vi "Align Mask and Signal - cluster.vi"(0 "Waveform":waveform(dbl)={"t0"=timestamp(0 s since 1904-01-01), "dt"=0.0, "Y"=[]}, 5 "trigger index":i32, 7 "upper limit":cluster{"x0":dbl, "dx":dbl, "Y":dbl[]} {"Y" format="%.2f"; "dx" format="%.2f"; "x0" format="%.2f"}, 9 "lower limit":cluster{"x0":dbl, "dx":dbl, "Y":dbl[]} {"Y" format="%.2f"; "dx" format="%.2f"; "x0" format="%.2f"}, 11 "error in (no error)":errorcluster, 12 "Mask Selector":u16(ring) items=["ITU", "EIA/TIA 547-1989"]) -> (3 "Subset Waveform":waveform(dbl), 4 "Waveform out":waveform(dbl), 6 "upper limit out":cluster{"x0":dbl, "dx":dbl, "Y":dbl[]} {"Y" format="%.2f"; "dx" format="%.2f"; "x0" format="%.2f"}, 8 "lower limit out":cluster{"x0":dbl, "dx":dbl, "Y":dbl[]} {"Y" format="%.2f"; "dx" format="%.2f"; "x0" format="%.2f"}, 15 "error out":errorcluster)   [LabVIEW 2012]
uses:
  <vilib>/Waveform/WDTOps.llb/WDT Number of Waveform Samples DBL.vi
  <vilib>/Waveform/WDTOps.llb/WDT Get Waveform Subset DBL (LV80).vi
  <vilib>/Waveform/WDTOps.llb/WDT Align Waveform Timestamps DBL.vi
  <vilib>/Analysis/NI_AALBase.lvlib
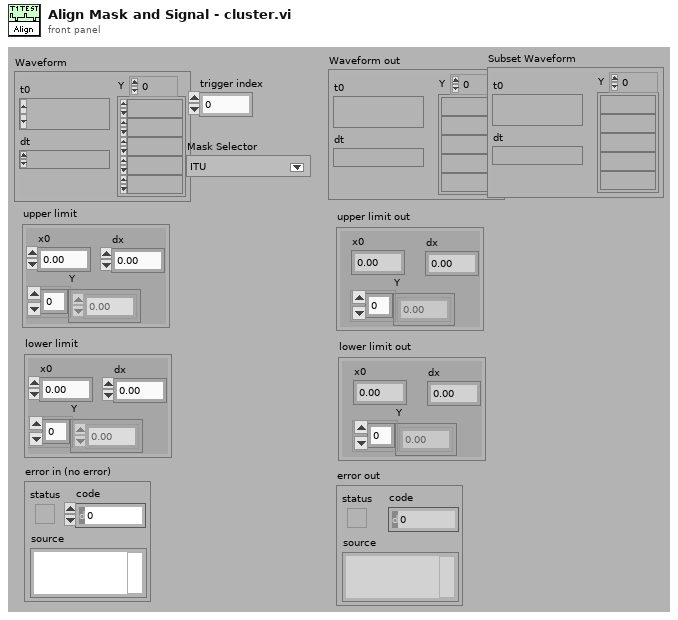
[diagram p1: front panel]
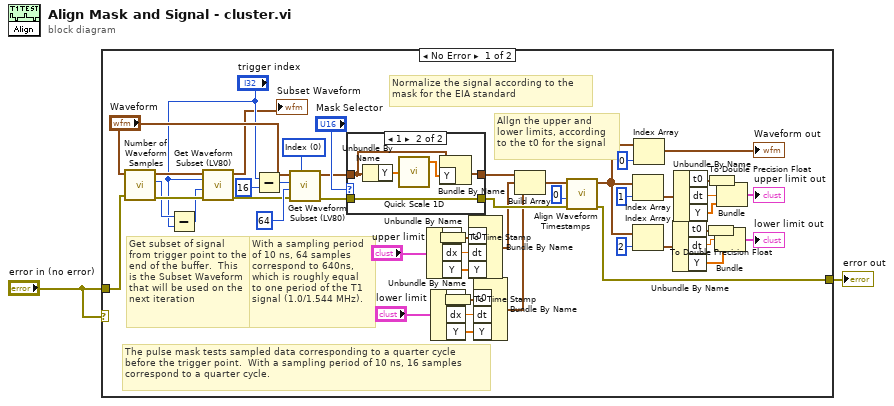
[diagram p0: block diagram]
diagram:
  n1 = case shown="No Error" "error in (no error)" {
    tunnel: "error in (no error)" -> [w39 w60]
    tunnel: [w45 w60] -> w1
    frame No Error {
      w40 = u16 0 items=["Index", "Relative Time"] ("Mode")
      # "Normalize the signal according to the \nmask for the EIA standard"
      # "Allgn the upper and \nlower limits, according \nto the t0 for the signal"
      # "The pulse mask tests sampled data corresponding to a quarter cycle\nbefore the trigger point.  With a sampling period of 10 ns, 16 samples \ncorrespond to a quarter cycle."
      # "With a sampling period\nof 10 ns, 64 samples\ncorrespond to 640ns, \nwhich is roughly equal \nto one period of the T1 \nsignal (1.0/1.544 MHz)."
      # "Get subset of signal\nfrom trigger point to the\nend of the buffer.  This\nis the Subset Waveform\nthat will be used on the \nnext iteration"
      n2 = call-poly <vilib>:"Number of Waveform Samples.vi"("error in (no error)"=w39, "waveform in"="Waveform") -> ("error out"=w37:errorcluster, "number of samples"=w35:i32, "waveform out"=w38:waveform(dbl))  [unwired: 7 in]
      n3 = Subtract(x=w35, y="trigger index") -> (x-y=w33:i32)
      n4 = call-poly <vilib>:"Get Waveform Subset (LV80).vi"("error in (no error)"=w37, "duration"=w33, "start samples/time"="trigger index", "waveform in"=w38) -> ("error out"=w36:errorcluster, "waveform out"=→"Subset Waveform":waveform(dbl))  [unwired: 2 in, 2 out]
      n5 = Subtract(x="trigger index", y=16) -> (x-y=w43:i32)
      n6 = call-poly <vilib>:"Get Waveform Subset (LV80).vi"("start/duration format"=w40, "error in (no error)"=w36, "duration"=64 ("Array Length"), "start samples/time"=w43, "waveform in"="Waveform") -> ("error out"=w30:errorcluster, "waveform out"=w28:waveform(dbl))  [unwired: 1 in, 2 out]
      n7 = case shown="1" "Mask Selector" {
        tunnel: w30 -> [w54 w59]
        tunnel: [w54 w59] -> w29
        tunnel: w28 -> [w53 w57]
        tunnel: [w53 w55] -> w27
        frame 0, Default {
        }
        frame 1 {
          n8 = Unbundle By Name(w57) -> ("Y"=w58:dbl[])
          n9 = call <vilib>:"Quick Scale 1D.vi"("X"=w58) -> ("Y[i]=X[i]/Max|X|"=w56:dbl[])  [unwired: 2 out]
          n10 = Bundle By Name(cluster=w57, "Y"=w56) -> (w55:waveform(dbl))
        }
      }
      n11 = Unbundle By Name("upper limit") -> ("x0"=w25:dbl, "dx"=w24:dbl, "Y"=w23:dbl[])
      n12 = Unbundle By Name("lower limit") -> ("x0"=w18:dbl, "dx"=w20:dbl, "Y"=w21:dbl[])
      n13 = To Time Stamp(1:w25) -> (0:w3:timestamp)
      n14 = To Time Stamp(1:w18) -> (0:w4:timestamp)
      n15 = Bundle By Name("t0"=w3, "dt"=w24, "Y"=w23) -> (w22:waveform(dbl))  [unwired: 1 in]
      n16 = Bundle By Name("t0"=w4, "dt"=w20, "Y"=w21) -> (w17:waveform(dbl))  [unwired: 1 in]
      n17 = Build Array(w27, w22, w17) -> (w52:waveform(dbl)[])
      n18 = call-poly <vilib>:"Align Waveform Timestamps.vi"("error in (no error)"=w29, "index"=0 ("Index"), "waveforms in"=w52) -> ("error out"=w45:errorcluster, "waveforms out"=w50:waveform(dbl)[])  [unwired: 7 in]
      n19 = Index Array(array=w50, index=1 ("Index")) -> (element=w16:waveform(dbl))
      n20 = Index Array(array=w50, index=2 ("Index")) -> (element=w11:waveform(dbl))
      n21 = Index Array(array=w50, index=0 ("Index")) -> (element=→"Waveform out":waveform(dbl))
      n22 = Unbundle By Name(w11) -> ("t0"=w6:timestamp, "dt"=w9:dbl, "Y"=w8:dbl[])
      n23 = Unbundle By Name(w16) -> ("t0"=w5:timestamp, "dt"=w14:dbl, "Y"=w13:dbl[])
      n24 = To Double Precision Float(number=w6) -> (double precision float=w10:dbl)
      n25 = To Double Precision Float(number=w5) -> (double precision float=w15:dbl)
      n26 = Bundle(w10, "dt"=w9, "Y"=w8) -> (→"lower limit out":cluster{dbl, "dt":dbl, "Y":dbl[]})  [unwired: 1 in]
      n27 = Bundle(w15, "dt"=w14, "Y"=w13) -> (→"upper limit out":cluster{dbl, "dt":dbl, "Y":dbl[]})  [unwired: 1 in]
    }
    frame Error {
    }
  }
  "error out" <- w1
